vi "StopOnSight_daryl_avg.vi"() -> ()   [LabVIEW 2013]
uses:
  <vilib>/Platform/TimedLoop/XDataNode/timing_clust.ctl
  <vilib>/Platform/TimedLoop/XDataNode/nitl_modes.ctl
  <vilib>/Platform/TimedLoop/XDataNode/wakeup.ctl
  <vilib>/Instr/_visa.llb/VISA Configure Serial Port (Instr).vi
  <vilib>/FPGAPlugInAG/sbRIO-9642/niLvFpga_Open_sbRIO-9642.vi
  <vilib>/rvi/interface/common/dynamic/niFpgaDynamicAddResources.vi
  <vilib>/rvi/interface/common/niFpgaWaitOnOcc.vi
  <vilib>/Utility/error.llb/Error Cluster From Error Code.vi
  <vilib>/rvi/errors/niLvFpgaAdjustHostInterfaceError.vi
  <vilib>/Platform/TimedLoop/XDataNode/XDataNode.xnode
  <vilib>/rvi/interface/nirviOpenFPGA/nirviOpenFPGA.xnode
  FPGA Bitfiles/NatesProject1_FPGATarget_FPGAConfig_gDHlPw7zMRU.lvbitx
  FPGA Config.vi
  <vilib>/rvi/interface/nirviReadWriteControl/nirviReadWriteControl.xnode
  <vilib>/Platform/TimedLoop/XDataNode/XDNodeRunTimeDep.lvlib
  NiFpgaLv.dll
  <vilib>/rvi/interface/Simulation/niFpgaSimulationCallBeginRW.vi
panel:
  out "i":fxp<+/-,32,32>
  in  "Avg Read":i32
  out "average":fxp<+/-,32,32>
  in  "Speed(%)":i32(knob) scale=0.0..100.0
  in  "Stop Distance":dbl(slide) scale=0.1..1.5
  out "error out":errorcluster
  out "Distance\n(cm)":dbl(slide) scale=0.0..2.5
  out "ModA/AI0":fxp<+/-,26,5>
  in  "VISA resource name":refnum<visa-resource-name>
  in  "stop":bool
  out "write buffer":string
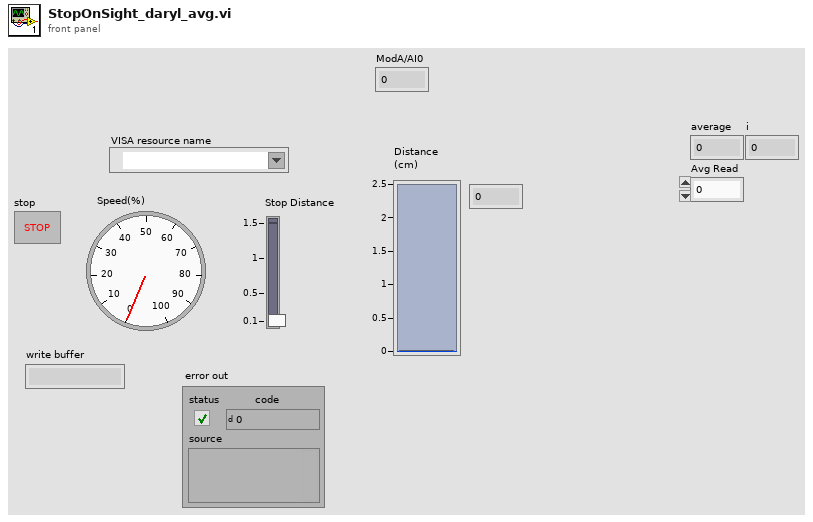
[diagram p1: front panel]
types:
  T1 = typedef "XDNodeRunTimeDep.lvlib/timing_clust.ctl" = cluster{"Expected End [f-1]":u64, "Actual End [f-1]":u64, "Finished Late? [f-1]":bool, "Expected End [i-1]":u64, "Actual End [i-1]":u64, "Finished Late? [i-1]":bool, "Expected Start [i]":u64, "Actual Start [i]":u64, "Expected Start [f]":u64, "Actual Start [f]":u64, "Source Name":string, "Structure Name":string, "Period":i64, "Deadline":i64, "Offset":i64, "Start":i64, "Priority":i32, "Timeout":i32, "Mode":T2, "Wakeup Reason":T3, "Error":errorcluster, "Source Type":string, "Secondary Source Type":string, "Global End Time":u64, "Global Start Time":u64, "Frame Duration":u64, "Iteration Duration":u64, "Assigned CPU":i32, "I/O Scan Engine Mode":u32}
  T2 = typedef "XDNodeRunTimeDep.lvlib/nitl_modes.ctl" = enum32{"No Change", "Process missed periods, maintain original phase", "Discard missed periods, maintain original phase", "Process missed periods, ignore original phase", "Discard missed periods, ignore original phase"}
  T3 = typedef "XDNodeRunTimeDep.lvlib/wakeup.ctl" = enum32{"Normal", "Aborted", "Asynchronous wakeup", "Timing source error", "Timed loop error", "Timeout"}
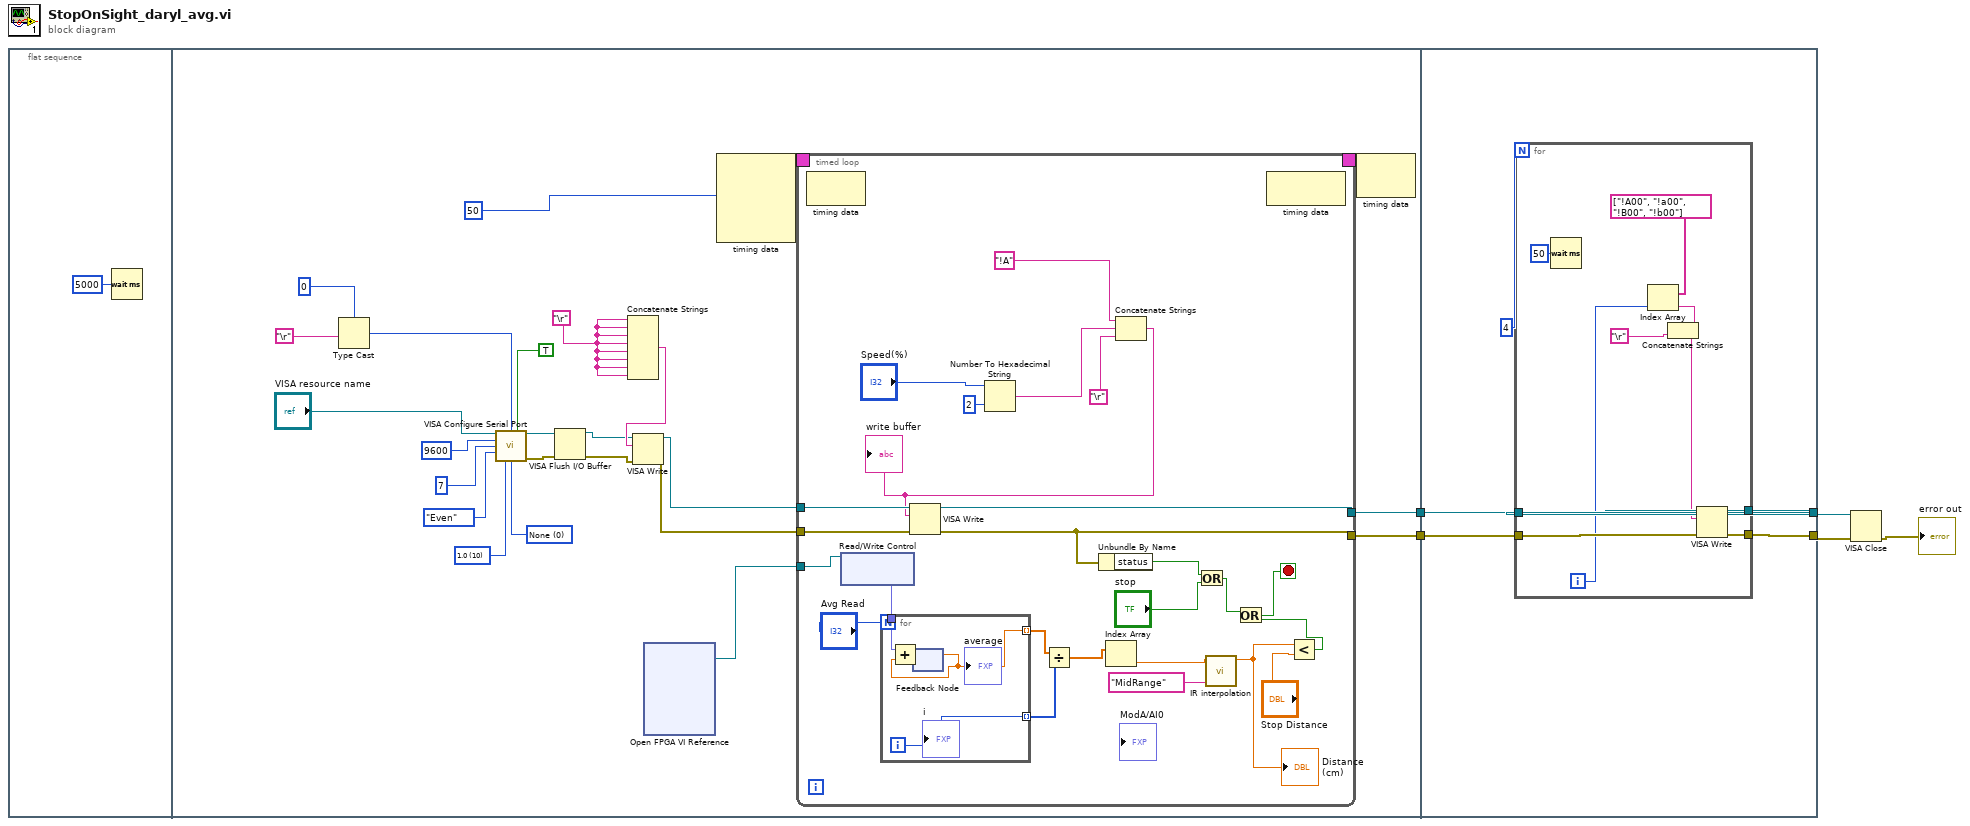
[diagram p0: block diagram]
diagram:
  n1 = flat-sequence {
    tunnel: [w9] -> w5
    tunnel: [w8] -> w4
    tunnel: [w67] -> w2
    tunnel: [w68] -> w3
    tunnel: w5 -> [w70]
    tunnel: w4 -> [w69]
    frame #0 {
      n2 = Wait (ms)(milliseconds to wait=u32 5000) -> ()  [unwired: 1 out]
    }
    frame #1 {
      w15 = "\r"
      w22 = u16 0 items=["None", "XON/XOFF", "RTS/CTS", "XON/XOFF & RTS/CTS", "DTR/DSR", "XON/XOFF & DTR/DSR"] ("flow control (0:none)")
      w23 = u16 10 items=["1.0"=10, "1.5"=15, "2.0"=20] ("stop bits (10: 1 bit)")
      n3 = Type Cast(type=0, x="\r") -> (*(type *) &x=w18:i32)
      n4 = call-poly "VISA Configure Serial Port"("VISA resource name"="VISA resource name", "termination char\n(0xA = '\\n' = LF)"=w18, "Enable Termination\nChar (T)"=TRUE ("Enable Termination\nChar (T)"), "baud rate (9600)"=u32 9600, "data bits (8)"=u16 7, "parity (0:none)"=enum16{"None", "Odd", "Even", "Mark", "Space"}."Even", "stop bits (10: 1 bit)"=w23, "flow control (0:none)"=w22) -> ("VISA resource name out"=w16:refnum<visa-resource-name>, "error out"=w17:errorcluster)  [unwired: 6 in]
      n5 = VISA Flush I/O Buffer(VISA resource name=w16, error in (no error)=w17) -> (VISA resource name out=w13:refnum<visa-resource-name>, error out=w12:errorcluster)  [unwired: 1 in]
      n6 = Concatenate Strings(w15, w15, w15, w15, w15, w15, w15, w15) -> (w14:string)
      n7 = VISA Write(VISA resource name=w13, write buffer=w14, error in (no error)=w12) -> (VISA resource name out=w11:refnum<visa-resource-name>, error out=w10:errorcluster)  [unwired: 1 out]
      n8 = xnode "Open FPGA VI Reference"() -> ("FPGA VI Reference Out"=w7:refnum<k20>)  [unwired: 2 in, 1 out]
      n9 = node-c288(i64 50 ("Period")) -> (w30:T1)  [unwired: 3 in]
      n10 = timed-loop {
        timing: w30 -> [_]
        timing-out: [_] -> w29
        tunnel: w11 -> [w52]
        tunnel: w10 -> [w51]
        tunnel: [w46] -> w9
        tunnel: [w47] -> w8
        tunnel: w7 -> [w42]
        stop <- w43 stop-if-true
        n11 = node-c288() -> ()  [unwired: 1 in, 1 out]
        n12 = xnode "Read/Write Control"("FPGA VI Reference In"=w42) -> ("ModA/AI1"=w36:fxp<+/-,26,5>)  [unwired: 1 in, 2 out]
        n13 = for {
          N: "Avg Read" -> [_]
          tunnel: w36 -> [w58]
          tunnel: [w57] -> w34 mode=indexing
          tunnel: [w56] -> w33 mode=indexing
          i -> [w56]
          n14 = feedback #1() -> (w57:dbl)  [unwired: 1 in]
          "average" <- w57
          n15 = Add(x=w58, y=w57) -> (x+y=w59:dbl)
          n16 = feedback-in #1(w59) -> ()
          "i" <- w56
        }
        n17 = Number To Hexadecimal String(1:i16 2 ("width (-)"), 2:"Speed(%)") -> (0:w54:string)
        n18 = Divide(x=w34, y=w33) -> (x/y=w32:dbl[])
        n19 = Index Array(array=w32) -> (element=w31:dbl)  [unwired: 1 in]
        n20 = Concatenate Strings("!A", w54, "\r") -> (w50:string)
        "write buffer" <- w50
        n21 = VISA Write(VISA resource name=w52, write buffer=w50, error in (no error)=w51) -> (VISA resource name out=w46:refnum<visa-resource-name>, error out=w47:errorcluster)  [unwired: 1 out]
        n22 = Unbundle By Name(w47) -> ("status"=w49:bool)
        n23 = Or(x=w49, y="stop") -> (x .or. y?=w44:bool)
        n24 = call "IR interpolation.vi"("IR Sensor Type"="MidRange", "x value"=w31) -> ("interpolation value"=w37:dbl)  [unwired: 9 in]
        "Distance\n(cm)" <- w37
        n25 = node-c288() -> ()  [unwired: 1 in, 1 out]
        n26 = Less?(x=w37, y="Stop Distance") -> (x < y?=w41:bool)
        n27 = Or(x=w44, y=w41) -> (x .or. y?=w43:bool)
      }
      n28 = node-c288(w29) -> ()  [unwired: 1 out]
    }
    frame #2 {
      n29 = for {
        N: 4 -> [_]
        tunnel: w70 -> [w80]
        tunnel: w69 -> [w79]
        tunnel: [w78] -> w68
        tunnel: [w77] -> w67
        i -> [w75]
        n30 = Wait (ms)(milliseconds to wait=u32 50) -> ()  [unwired: 1 out]
        n31 = Index Array(array=string[] ["!A00", "!a00", "!B00", "!b00"], index=w75) -> (element=w73:string)
        n32 = Concatenate Strings(w73, "\r") -> (w71:string)
        n33 = VISA Write(VISA resource name=w80, write buffer=w71, error in (no error)=w79) -> (VISA resource name out=w78:refnum<visa-resource-name>, error out=w77:errorcluster)  [unwired: 1 out]
      }
    }
  }
  n34 = VISA Close(VISA resource name=w3, error in (no error)=w2) -> (error out=→"error out":errorcluster)
